vi "CritOpal.vi"() -> ()   [LabVIEW 2014]
uses:
  Instance           2 23Saved   Vvstime-new-new .vi
  Instance           3 23Saved   Vvstime-new-new .vi
panel:
  in  "Voltmeter 2 address":string="22"
  out "XY Graph 2":cluster{dbl[], dbl[]}[](graph)=[{[4.266361713409424, 29.083149433135986, 43.507516860961914, 56.900455474853516, 70.34027767181396, 91.54706621170044, 109.03446292877197, 124.52151346206665, 139.9773087501526], [0.0, 0.0, 0.0, 0.0, 0.0, 0.0, 0.0, 0.0, 0.0]}, {[4.266361713409424, 29.083149433135986, 43.507516860961914, 56.900455474853516, 70.34027767181396, 91.54706621170044, 109.03446292877197, 124.52151346206665, 139.9773087501526], [28.709, 28.728, 28.754, 28.777, 28.811, 28.838, 28.865, 28.891, 28.922]}]
  out "XY Graph":cluster{dbl[], dbl[]}[](graph)=[{[4.266361713409424, 29.083149433135986, 43.507516860961914, 56.900455474853516, 70.34027767181396, 91.54706621170044, 109.03446292877197, 124.52151346206665, 139.9773087501526], [10517.0, 10517.0, 10519.0, 10517.0, 10518.0, 10515.0, 10512.0, 10510.0, 10517.0]}, {[4.266361713409424, 29.083149433135986, 43.507516860961914, 56.900455474853516, 70.34027767181396, 91.54706621170044, 109.03446292877197, 124.52151346206665, 139.9773087501526], [29.512, 29.643, 29.762, 29.805, 0.0, 29.866, 29.892, 29.911, 29.942]}]
  in  "Voltmeter 1 address":string="11"
  in  "Sample Temp Address":string="15"
  in  "Wait (s)":dbl=3.0 format="%.2f"
  in  "Start/Stop":bool=TRUE
  in  "File Name":string="testing"
  # "Critical Opalescence"
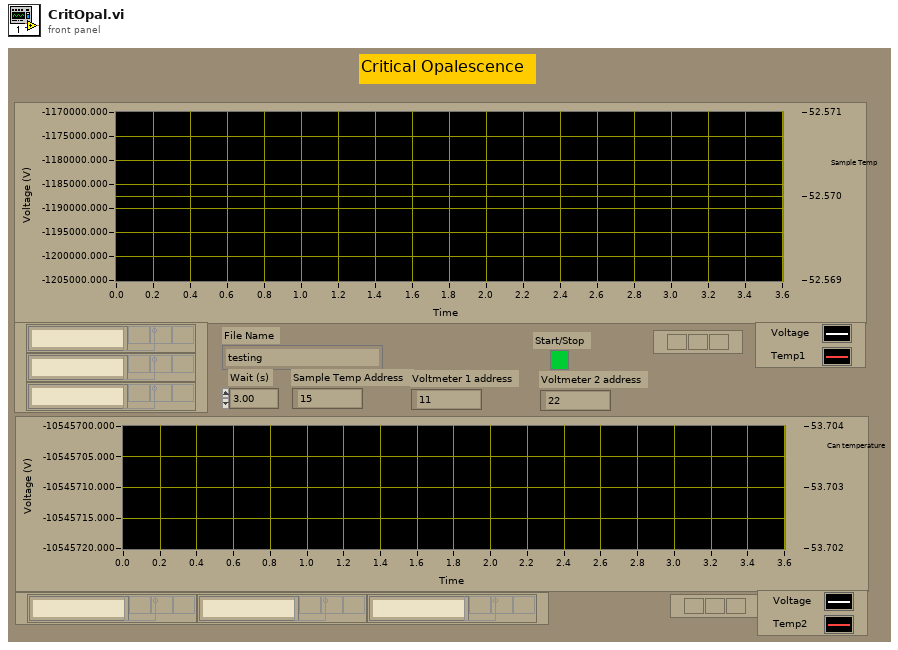
[diagram p1: front panel]
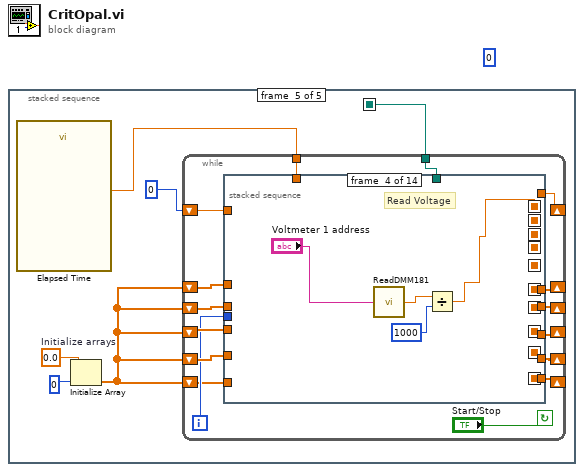
[diagram p0: block diagram]
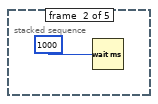
[diagram p3: hidden frame]
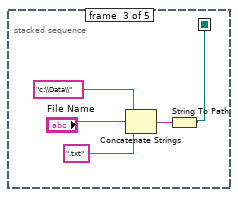
[diagram p4: hidden frame]
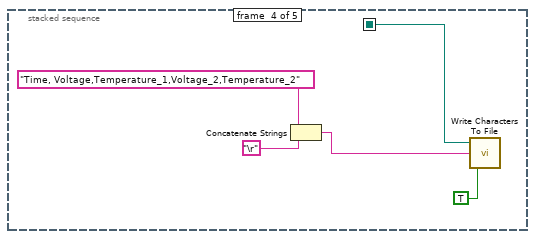
[diagram p5: hidden frame]
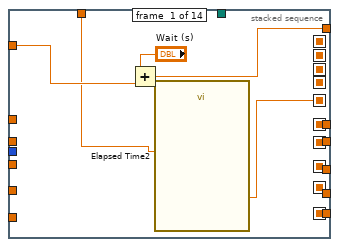
[diagram p6: hidden frame]
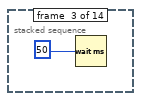
[diagram p8: hidden frame]
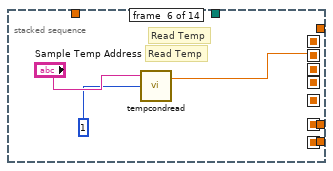
[diagram p10: hidden frame]
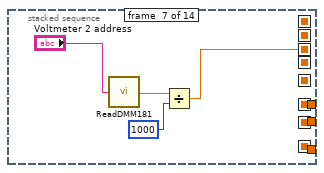
[diagram p11: hidden frame]
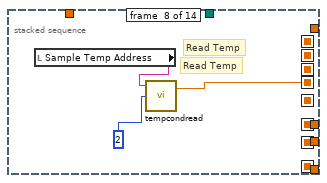
[diagram p12: hidden frame]
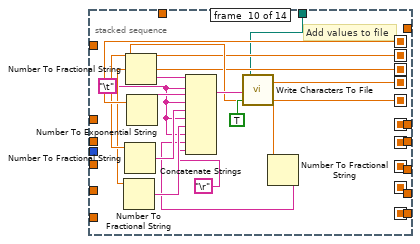
[diagram p14: hidden frame]
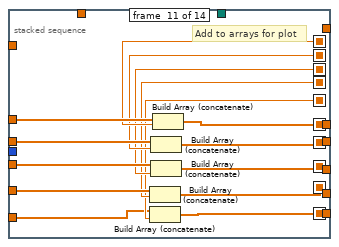
[diagram p15: hidden frame]
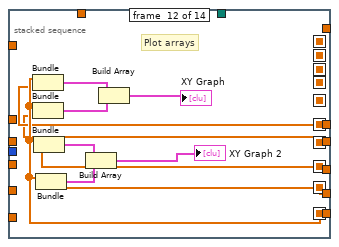
[diagram p16: hidden frame]
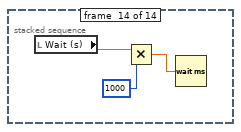
[diagram p18: hidden frame]
diagram:
  (unwired) 0
  n1 = stacked-sequence {
    seq-local: [_ _ w2 _ _] -> [_ _ _ w7 w14]
    frame #0 {
      # "init devices"
    }
    frame #1 {
      n2 = Wait (ms)(milliseconds to wait=1000) -> ()  [unwired: 1 out]
    }
    frame #2 {
      n3 = Concatenate Strings("c:\\Data\\", "File Name", ".txt") -> (w3:string)
      n4 = String To Path(string=w3) -> (path=w2:path)
    }
    frame #3 {
      n5 = Concatenate Strings("Time, Voltage,Temperature_1,Voltage_2,Temperature_2", "\r") -> (w8:string)
      n6 = call <vilib>:"Write Characters To File.vi"("append to file? (new file:F)"=TRUE, "character string"=w8, "file path (dialog if empty)"=w7) -> ()  [unwired: 2 in, 1 out]
    }
    frame #4 {
      w17 = 0.0  # Initialize arrays
      n7 = call "Elapsed Time"() -> ("Get Start Time (s)"=w12:dbl)  [unwired: 12 in, 7 out]
      n8 = Initialize Array(w17, 0) -> (w15:dbl[])
      n9 = while {
        tunnel: w14 -> [w19]
        shift-left: 0 -> [w21]
        shift-right: [w20] -> _
        shift-left: w15 -> [w23]
        shift-right: [w22] -> _
        shift-left: w15 -> [w27]
        shift-right: [w25] -> _
        shift-left: w15 -> [w28]
        shift-right: [w24] -> _
        shift-left: w15 -> [w32]
        shift-right: [w30] -> _
        shift-left: w15 -> [w33]
        shift-right: [w31] -> _
        tunnel: w12 -> [w18]
        i -> [w26]
        stop <- "Start/Stop" continue-if-true
        n10 = stacked-sequence {
          seq-local: [_ _ _ _ _ w44 _ _ _ _ _ _ _ _] -> [_ _ _ _ _ _ _ _ _ w62 w74 _ _ _]
          seq-local: [w35 _ _ _ _ _ _ _ _ _ _ _ _ _] -> [_ _ _ _ _ _ _ _ _ w64 w71 _ _ _]
          seq-local: [_ _ _ _ _ _ _ _ _ _ w81 _ _ _] -> [_ _ _ _ _ _ _ _ _ _ _ w92 _ _]
          seq-local: [_ _ _ _ _ _ _ _ _ _ w80 _ _ _] -> [_ _ _ _ _ _ _ _ _ _ _ w91 _ _]
          seq-local: [_ _ _ _ _ _ _ _ _ _ w77 _ _ _] -> [_ _ _ _ _ _ _ _ _ _ _ w94 _ _]
          seq-local: [_ _ _ _ _ _ _ _ _ _ w76 _ _ _] -> [_ _ _ _ _ _ _ _ _ _ _ w86 _ _]
          seq-local: [_ _ _ w41 _ _ _ _ _ _ _ _ _ _] -> [_ _ _ _ _ _ _ _ _ w63 w75 _ _ _]
          seq-local: [_ _ _ _ _ _ w47 _ _ _ _ _ _ _] -> [_ _ _ _ _ _ _ _ _ w61 w73 _ _ _]
          seq-local: [_ _ _ _ _ _ _ w51 _ _ _ _ _ _] -> [_ _ _ _ _ _ _ _ _ w58 w72 _ _ _]
          seq-local: [_ _ _ _ _ _ _ _ _ _ w69 _ _ _] -> [_ _ _ _ _ _ _ _ _ _ _ w93 _ _]
          tunnel: w33 -> [_ _ _ _ _ _ _ _ _ _ w83 _ _ _]
          tunnel: w32 -> [_ _ _ _ _ _ _ _ _ _ w82 _ _ _]
          tunnel: [_ _ _ _ _ _ _ _ _ _ w81 _ _ _] -> w31
          tunnel: [_ _ _ _ _ _ _ _ _ _ w80 _ _ _] -> w30
          tunnel: w26 -> [_ _ _ _ _ _ _ _ _ _ _ _ _ _]
          tunnel: w28 -> [_ _ _ _ _ _ _ _ _ _ w79 _ _ _]
          tunnel: w27 -> [_ _ _ _ _ _ _ _ _ _ w78 _ _ _]
          tunnel: [_ _ _ _ _ _ _ _ _ _ _ w86 _ _] -> w25
          tunnel: [_ _ _ _ _ _ _ _ _ _ _ w94 _ _] -> w24
          tunnel: w21 -> [w36 _ _ _ _ _ _ _ _ _ _ _ _ _]
          tunnel: [w38 _ _ _ _ _ _ _ _ _ _ _ _ _] -> w20
          tunnel: w23 -> [_ _ _ _ _ _ _ _ _ _ w70 _ _ _]
          tunnel: [_ _ _ _ _ _ _ _ _ _ w69 _ _ _] -> w22
          tunnel: w19 -> [_ _ _ _ _ _ _ _ _ w55 _ _ _ _]
          tunnel: w18 -> [w34 _ _ _ _ _ _ _ _ _ _ _ _ _]
          frame #0 {
            n11 = Add(x="Wait (s)", y=w36) -> (x+y=w38:dbl)
            n12 = call "Elapsed Time2"("Set Start Time (s)"=w34) -> ("Elapsed Time (s)"=w35:dbl)  [unwired: 11 in, 7 out]
          }
          frame #1 {
          }
          frame #2 {
            n13 = Wait (ms)(milliseconds to wait=50) -> ()  [unwired: 1 out]
          }
          frame #3 {
            # "Read Voltage"
            n14 = call "ReadDMM181.vi"("DMM GPIB Address"="Voltmeter 1 address") -> ("DMM read (mV)"=w40:dbl)
            n15 = Divide(x=w40, y=1000) -> (x/y=w41:dbl)
          }
          frame #4 {
          }
          frame #5 {
            # "Read Temp"
            # "Read Temp"
            n16 = call "tempcondread.vi"("Ring"=1, "GPIB Address"="Sample Temp Address") -> ("Temperature"=w44:dbl)  [unwired: 1 in, 1 out]
          }
          frame #6 {
            n17 = call "ReadDMM181.vi"("DMM GPIB Address"="Voltmeter 2 address") -> ("DMM read (mV)"=w49:dbl)
            n18 = Divide(x=w49, y=1000) -> (x/y=w47:dbl)
          }
          frame #7 {
            # "Read Temp"
            # "Read Temp"
            n19 = local read "Sample Temp Address"() -> (w53:string)
            n20 = call "tempcondread.vi"("Ring"=2, "GPIB Address"=w53) -> ("Temperature"=w51:dbl)  [unwired: 1 in, 1 out]
          }
          frame #8 {
          }
          frame #9 {
            w56 = "\t"
            # "Add values to file"
            n21 = Number To Fractional String(number=w61) -> (F-format string=w60:string)  [unwired: 3 in]
            n22 = Number To Fractional String(number=w62) -> (F-format string=w65:string)  [unwired: 3 in]
            n23 = Number To Fractional String(number=w64) -> (F-format string=w68:string)  [unwired: 3 in]
            n24 = Number To Exponential String(number=w63) -> (E-format string=w57:string)  [unwired: 3 in]
            n25 = Number To Fractional String(number=w58) -> (F-format string=w59:string)  [unwired: 3 in]
            n26 = Concatenate Strings(w68, w56, w57, w56, w65, w56, w60, w56, w59, "\r") -> (w66:string)
            n27 = call <vilib>:"Write Characters To File.vi"("append to file? (new file:F)"=TRUE, "character string"=w66, "file path (dialog if empty)"=w55) -> ()  [unwired: 2 in, 1 out]
          }
          frame #10 {
            # "Add to arrays for plot"
            n28 = Build Array (concatenate)(w78, w72) -> (w76:dbl[])
            n29 = Build Array (concatenate)(w70, w71) -> (w69:dbl[])
            n30 = Build Array (concatenate)(w82, w74) -> (w80:dbl[])
            n31 = Build Array (concatenate)(w79, w73) -> (w77:dbl[])
            n32 = Build Array (concatenate)(w83, w75) -> (w81:dbl[])
          }
          frame #11 {
            # "Plot arrays"
            n33 = Bundle(w93, w92) -> (w90:cluster{dbl[], dbl[]})  [unwired: 1 in]
            n34 = Bundle(w93, w91) -> (w89:cluster{dbl[], dbl[]})  [unwired: 1 in]
            n35 = Bundle(w93, w94) -> (w88:cluster{dbl[], dbl[]})  [unwired: 1 in]
            n36 = Bundle(w93, w86) -> (w87:cluster{dbl[], dbl[]})  [unwired: 1 in]
            n37 = Build Array(w88, w87) -> (→"XY Graph 2":cluster{dbl[], dbl[]}[])
            n38 = Build Array(w90, w89) -> (→"XY Graph":cluster{dbl[], dbl[]}[])
          }
          frame #12 {
          }
          frame #13 {
            n39 = local read "Wait (s)"() -> (w95:dbl)
            n40 = Multiply(x=w95, y=1000) -> (x*y=w96:dbl)
            n41 = Wait (ms)(milliseconds to wait=w96) -> ()  [unwired: 1 out]
          }
        }
      }
    }
  }
